vi "ingest.tabular_set_timestamp_custom.vi"(8 "error in":errorcluster, 11 "TabularIngestStaging in":refnum<class "TabularIngestStaging.lvclass">) -> (0 "error out":errorcluster, 3 "TabularIngestStaging out":refnum<class "TabularIngestStaging.lvclass">)   [LabVIEW 2020, in "TabularIngestStaging.lvclass"]
doc: "Specifies that row timestamps use a custom date/time format in the named column."
uses:
  TabularIngestStaging.lvclass
  TabularIngestStaging.lvclass/TabularIngestStaging.ctl
  client.lvlib
panel:
  in  "column":string
  in  "format":string
  in  "default_year":i32
  in  "default_day_of_year":i32
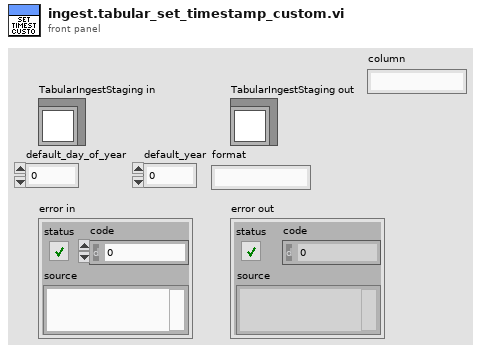
[diagram p1: front panel]
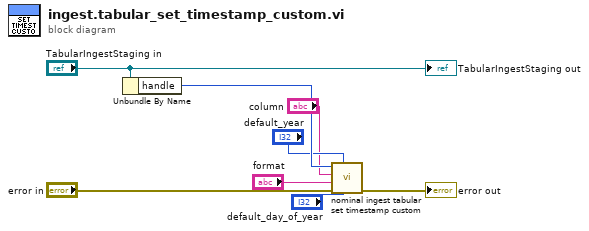
[diagram p0: block diagram]
diagram:
  n1 = Unbundle By Name("TabularIngestStaging in") -> ("handle"=w6:i32)
  n2 = call "nominal ingest tabular set timestamp custom.vi"("default_day_of_year"="default_day_of_year", "default_year"="default_year", "error in (no error)"="error in", "format"="format", "column"="column", "staging"=w6) -> ("error out"=→"error out":errorcluster)  [unwired: 4 in, 1 out]
  "TabularIngestStaging out" <- "TabularIngestStaging in"
